vi "rqcBob ServiceNET Check Connection.vi"(8 "error in":errorcluster, 11 "rqcBob ServiceNET in":T1) -> (0 "error out":errorcluster, 3 "rqcBob ServiceNET out":T1)   [LabVIEW 2018]
uses:
  Custom Controls/rqcBob ServiceNET control.ctl
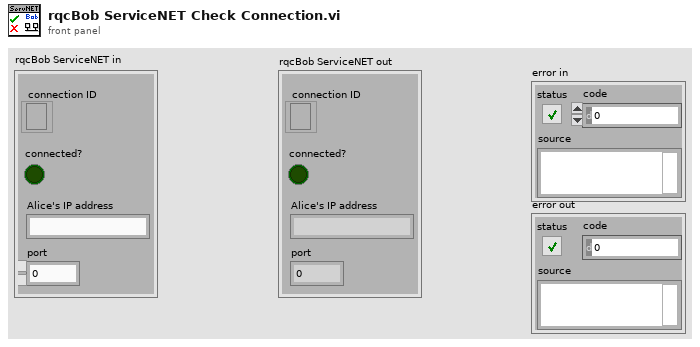
[diagram p1: front panel]
types:
  T1 = typedef "rqcBob ServiceNET control.ctl" = cluster{"connection ID":refnum<k5>, "connected?":bool, "Alice's IP address":string, "port":u16}
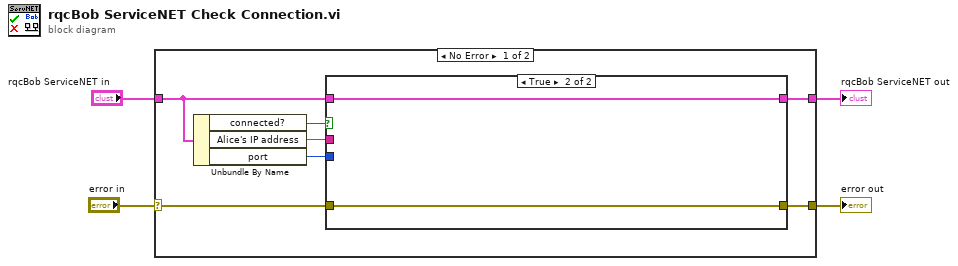
[diagram p0: block diagram]
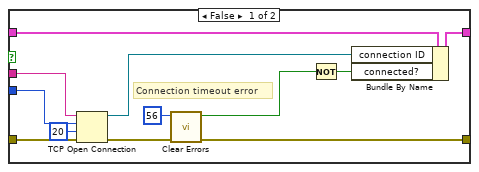
[diagram p2: hidden frame]
diagram:
  n1 = case shown="No Error" "error in" {
    selector: "error in" -> [w9 w27]
    tunnel: "rqcBob ServiceNET in" -> [w10 w26]
    tunnel: [w6 w27] -> w2
    tunnel: [w5 w26] -> w1
    frame No Error {
      n2 = Unbundle By Name(w10) -> ("connected?"=w11:bool, "Alice's IP address"=w8:string, "port"=w7:u16)
      n3 = case shown="True" w11 {
        tunnel: w10 -> [w19 w24]
        tunnel: w9 -> [w23 w25]
        tunnel: w8 -> [w22 _]
        tunnel: w7 -> [w21 _]
        tunnel: [w16 w25] -> w6
        tunnel: [w12 w24] -> w5
        frame False {
          # "Connection timeout error"
          n4 = TCP Open Connection(address=w22, remote port or service name=w21, timeout ms (60000)=20, error in (no error)=w23) -> (connection ID=w17:refnum<k5>, error out=w18:errorcluster)  [unwired: 1 in]
          n5 = call <vilib>:"Clear Errors.vi"("error in (no error)"=w18, "specific error code to clear (0: all)"=56) -> ("error out"=w16:errorcluster, "specific error cleared?"=w14:bool)  [unwired: 4 in]
          n6 = Not(x=w14) -> (.not. x?=w13:bool)
          n7 = Bundle By Name(cluster=w19, "connection ID"=w17, "connected?"=w13) -> (w12:T1)
        }
        frame True {
        }
      }
    }
    frame Error {
    }
  }
  "error out" <- w2
  "rqcBob ServiceNET out" <- w1
